vi "Run.vi"(8 "error in (no error)":errorcluster, 11 "FitterBase in":refnum<class "FitterBase.lvclass">) -> (0 "error out":errorcluster, 2 "TimeOut":bool, 3 "FitterBase out":refnum<class "FitterBase.lvclass">)   [LabVIEW 2014, in "AnalysisPlugins.lvlib" / "FitterBase.lvclass"]
uses:
  FitterBase.lvclass
  AnalysisPluginBaseClass/AnalysisPluginsBase.lvclass/AnalysisPluginsBase.ctl
  AnalysisPluginBaseClass/Accessors/Read SensorQue.vi
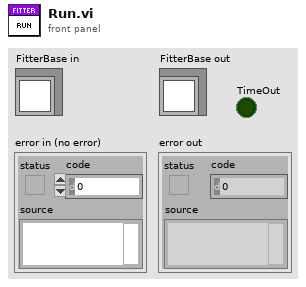
[diagram p1: front panel]
types:
  T1 = typedef "AnalysisPlugins.lvlib/AnalysisPluginsBase.lvclass/clSensorData.ctl" = cluster{"SensorType":string, "SensorData":variant}
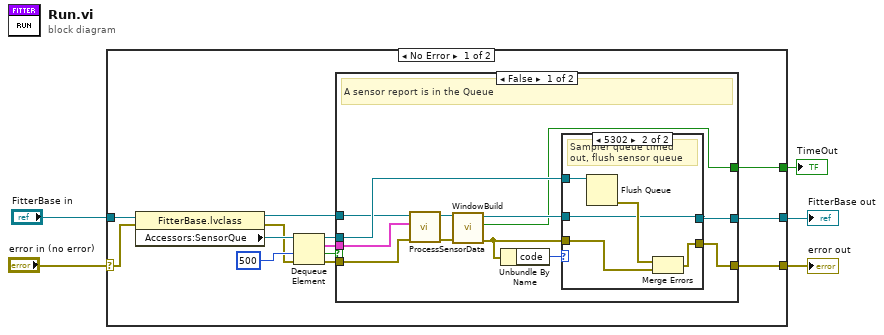
[diagram p0: block diagram]
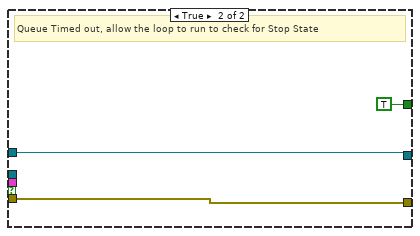
[diagram p3: hidden frame]
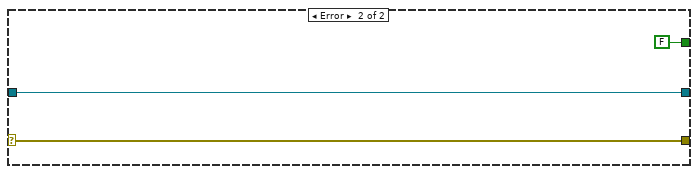
[diagram p4: hidden frame]
diagram:
  n1 = case shown="No Error" "error in (no error)" {
    selector: "error in (no error)" -> [w17 w42]
    tunnel: "FitterBase in" -> [w18 w43]
    tunnel: [w8 w43] -> w1
    tunnel: [w7 w42] -> w3
    tunnel: [w6 FALSE] -> w2
    frame No Error {
      n2 = property class="FitterBase.lvclass"(reference=w18, error in=w17) -> (reference out=w9:refnum<class "FitterBase.lvclass">, error out=w14:errorcluster, "Accessors:SensorQue"=w16:refnum<queue>)
      n3 = Dequeue Element(queue=w16, timeout in ms (-1)=500, error in (no error)=w14) -> (queue out=w13:refnum<queue>, element=w10:T1, timed out?=w11:bool, error out=w12:errorcluster)
      n4 = case shown="False" w11 {
        tunnel: w10 -> [w28 _]
        tunnel: w12 -> [w30 w40]
        tunnel: [w25 w40] -> w7
        tunnel: w13 -> [w24 _]
        tunnel: w9 -> [w21 w39]
        tunnel: [w20 w39] -> w8
        tunnel: [w19 TRUE] -> w6
        frame False {
          # "A sensor report is in the Queue"
          n5 = call-dynamic "ProcessSensorData.vi"("error in (no error)"=w30, "clSensorData"=w28, "Class In"=w21) -> ("error out"=w22:errorcluster, "Class Out"=w23:refnum<class "FitterBase.lvclass">)  [unwired: 7 in]
          n6 = call "WindowBuild.vi"("error in (no error)"=w22, "Fitter in"=w23) -> ("error out"=w26:errorcluster, "Timeout"=w19:bool, "Fitter out"=w27:refnum<class "FitterBase.lvclass">)  [unwired: 7 in]
          n7 = Unbundle By Name(w26) -> ("code"=w29:i32)
          n8 = case shown="5302" w29 {
            tunnel: w27 -> [w32 w33]
            tunnel: w26 -> [w31 w34]
            tunnel: [w31 w37] -> w25
            tunnel: w24 -> [_ w36]
            tunnel: [w32 w33] -> w20
            frame 0, Default {
            }
            frame 5302 {
              # "Sampler queue timed out, flush sensor queue"
              n9 = Flush Queue(queue=w36) -> (error out=w35:errorcluster)  [unwired: 1 in, 2 out]
              n10 = Merge Errors(w35, w34) -> (w37:errorcluster)
            }
          }
        }
        frame True {
          # "Queue Timed out, allow the loop to run to check for Stop State"
        }
      }
    }
    frame Error {
    }
  }
  "error out" <- w3
  "FitterBase out" <- w1
  "TimeOut" <- w2
